vi "Read States.vi"(8 "error in (no error)":errorcluster, 11 "BallPlacementEnemyTactic in":refnum<class "BallPlacementEnemyTactic.lvclass">) -> (0 "error out":errorcluster, 2 "States":T1, 3 "BallPlacementEnemyTactic out":refnum<class "BallPlacementEnemyTactic.lvclass">)   [LabVIEW 2023, in "BallPlacementEnemyTactic.lvclass"]
uses:
  BallPlacementEnemyTactic.lvclass
  StatesBallPlacementEnemyTactic.ctl
  BallPlacementEnemyTactic.lvclass/BallPlacementEnemyTactic.ctl
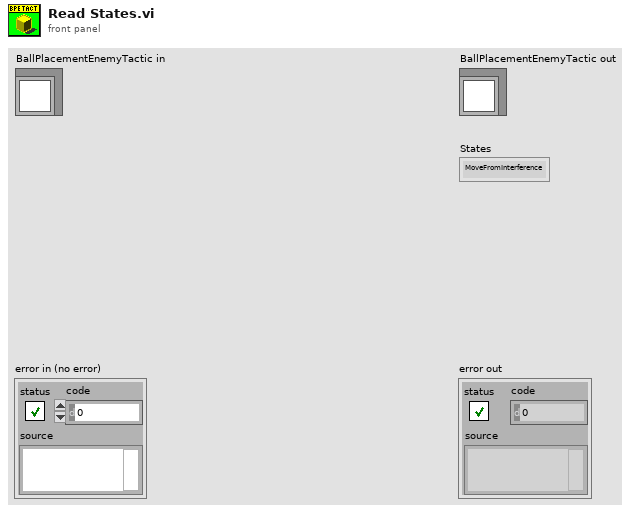
[diagram p1: front panel]
types:
  T1 = typedef "BallPlacementEnemyTactic.lvclass/StatesBallPlacementEnemyTactic.ctl" = enum16{"MoveFromInterference", "Halt", "Exit"}
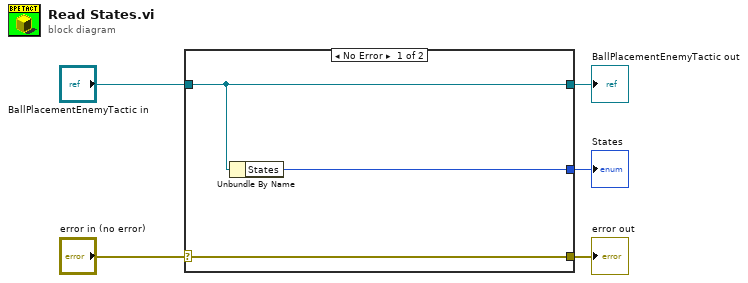
[diagram p0: block diagram]
diagram:
  n1 = case shown="No Error" "error in (no error)" {
    selector: "error in (no error)" -> [w8 w9]
    tunnel: [w8 w9] -> w4
    tunnel: [w7 w10] -> w2
    tunnel: "BallPlacementEnemyTactic in" -> [w7 w10]
    tunnel: [w6 _] -> w1
    frame No Error {
      n2 = Unbundle By Name(w7) -> ("States"=w6:T1)
    }
    frame Error {
    }
  }
  "error out" <- w4
  "BallPlacementEnemyTactic out" <- w2
  "States" <- w1
